vi "Send LimitOverride Event.vi"(8 "error in (no error)":errorcluster, 10 "event data":dbl, 11 "SignalWithAlarm in":refnum<class "SignalWithAlarm.lvclass">) -> (0 "error out":errorcluster, 3 "SignalWithAlarm out":refnum<class "SignalWithAlarm.lvclass">)   [LabVIEW 2016, in "SignalWithAlarm.lvclass"]
uses:
  SignalWithAlarm.lvclass
  SignalWithAlarm.lvclass/SignalWithAlarm.ctl
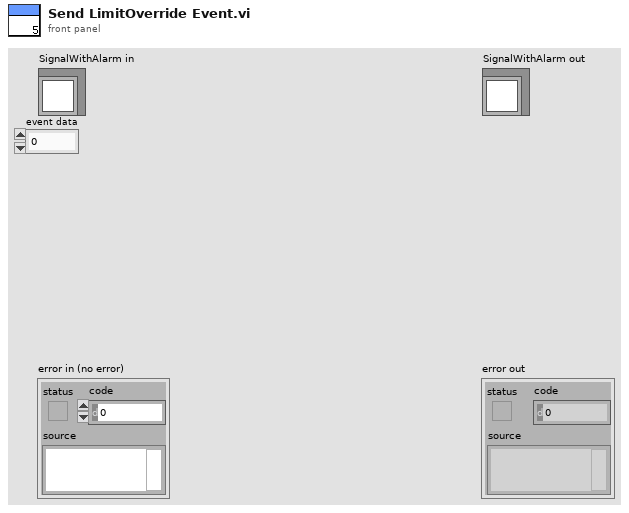
[diagram p1: front panel]
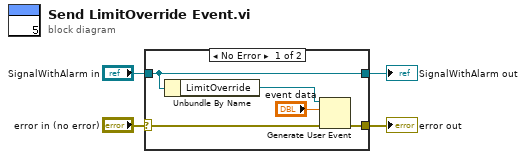
[diagram p0: block diagram]
diagram:
  n1 = case shown="No Error" "error in (no error)" {
    selector: "error in (no error)" -> [w6 w11]
    tunnel: [w5 w11] -> w3
    tunnel: [w9 w10] -> w1
    tunnel: "SignalWithAlarm in" -> [w9 w10]
    frame No Error {
      n2 = Unbundle By Name(w9) -> ("LimitOverride"=w8:refnum<user-event>)
      n3 = Generate User Event(user event=w8, event data cluster="event data", error in=w6) -> (error out=w5:errorcluster)  [unwired: 1 in, 1 out]
    }
    frame Error {
    }
  }
  "error out" <- w3
  "SignalWithAlarm out" <- w1
